vi "GetSelection1.vi"(1 "WFGraph Refnum":refnum<vi>) -> (0 "range":cluster{"x0":dbl, "x1":dbl} {"x1" format="%.2f"; "x0" format="%.2f"})   [LabVIEW 2009]
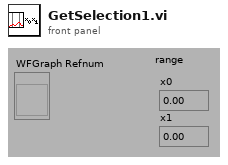
[diagram p1: front panel]
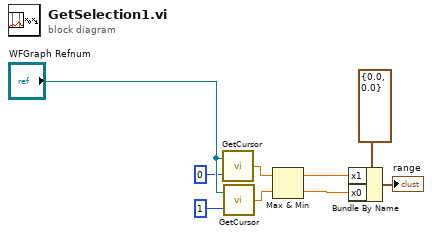
[diagram p0: block diagram]
diagram:
  n1 = call "GetCursor.vi"("Active Cursor"=u32 0, "WFGraph Refnum"="WFGraph Refnum") -> ("Cursor.Cursor X"=w5:dbl)
  n2 = call "GetCursor.vi"("Active Cursor"=u32 1, "WFGraph Refnum"="WFGraph Refnum") -> ("Cursor.Cursor X"=w9:dbl)
  n3 = Max & Min(x=w5, y=w9) -> (max(x,y)=w3:dbl, min(x,y)=w2:dbl)
  n4 = Bundle By Name(cluster=cluster{"x0":dbl, "x1":dbl} {"x0"=0.0, "x1"=0.0}, "x1"=w3, "x0"=w2) -> (→"range":cluster{"x0":dbl, "x1":dbl})
